vi "Read Asynchronous Measurement (Current and Voltage).vi"(6 "Wait Time (10 S)":u32=10, 7 "Voltage Buffer (smua.nvbuffer2)":string="smua.nvbuffer2", 8 "error in (no error)":errorcluster, 9 "Current Buffer (smua.nvbuffer1)":string="smua.nvbuffer1", 10 "Source Measure Unit Channel (0: Channel A)":i32(ring) items=["Channel A", "Channel B"], 11 "VISA resource name":refnum<visa-resource-name>) -> (0 "error out":errorcluster, 1 "Voltage Buffer Data (V)":dbl[](array[numeric]), 2 "Current Buffer Data (A)":dbl[](array[numeric]), 3 "VISA resource name out":refnum<visa-resource-name>)   [LabVIEW 2020, in "Keithley 2600 Series.lvlib"]
doc: "Returns the asynchronous current and voltage measurements."
uses:
  <instrlib>/Keithley 2600 Series/Keithley 2600 Series.lvlib
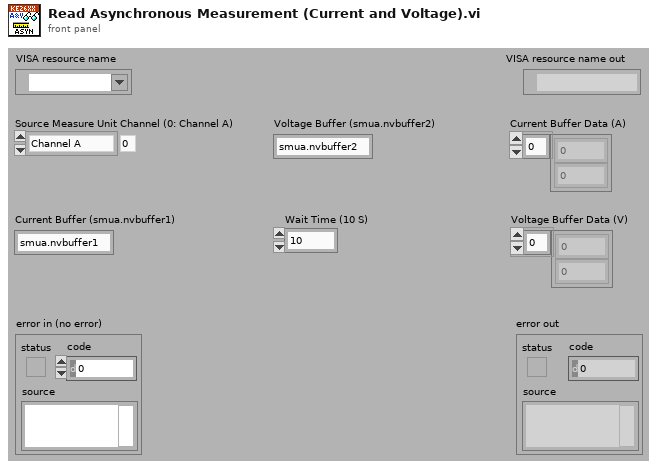
[diagram p1: front panel]
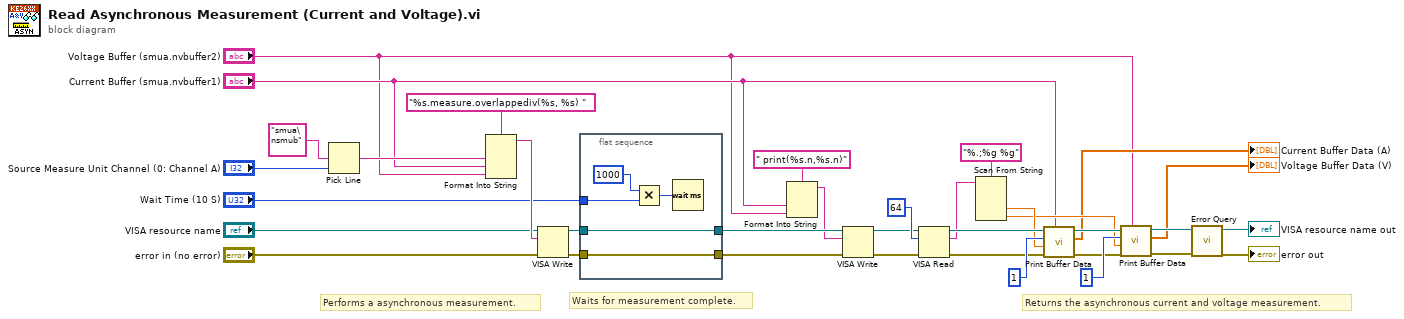
[diagram p0: block diagram]
diagram:
  # "Performs a asynchronous measurement."
  # "Waits for measurement complete."
  # "Returns the asynchronous current and voltage measurement."
  n1 = Pick Line(multi-line string="smua\nsmub", line index="Source Measure Unit Channel (0: Channel A)") -> (output string=w27:string)  [unwired: 1 in]
  n2 = Format Into String(format string="%s.measure.overlappediv(%s, %s) ", w27, "Current Buffer (smua.nvbuffer1)", "Voltage Buffer (smua.nvbuffer2)") -> (resulting string=w34:string)  [unwired: 2 in, 1 out]
  n3 = VISA Write(VISA resource name="VISA resource name", write buffer=w34, error in (no error)="error in (no error)") -> (VISA resource name out=w11:refnum<visa-resource-name>, error out=w10:errorcluster)  [unwired: 1 out]
  n4 = flat-sequence {
    tunnel: w11 -> [w40]
    tunnel: [w40] -> w8
    tunnel: [w39] -> w7
    tunnel: w10 -> [w39]
    tunnel: "Wait Time (10 S)" -> [w38]
    frame #0 {
      n5 = Multiply(x=u32 1000, y=w38) -> (x*y=w36:u32)
      n6 = Wait (ms)(milliseconds to wait=w36) -> ()  [unwired: 1 out]
    }
  }
  n7 = Format Into String(format string=" print(%s.n,%s.n)", "Current Buffer (smua.nvbuffer1)", "Voltage Buffer (smua.nvbuffer2)") -> (resulting string=w1:string)  [unwired: 2 in, 1 out]
  n8 = VISA Write(VISA resource name=w8, write buffer=w1, error in (no error)=w7) -> (VISA resource name out=w6:refnum<visa-resource-name>, error out=w5:errorcluster)  [unwired: 1 out]
  n9 = VISA Read(VISA resource name=w6, byte count=u32 64, error in (no error)=w5) -> (VISA resource name out=w24:refnum<visa-resource-name>, read buffer=w22:string, error out=w23:errorcluster)  [unwired: 1 out]
  n10 = Scan From String(format string="%.;%g %g", input string=w22) -> (output 1=w21:dbl, output 2=w14:dbl)  [unwired: 4 in, 3 out]
  n11 = call <instrlib>:"Print Buffer Data.vi"("Reading Buffer (smua.nvbuffer1)"="Current Buffer (smua.nvbuffer1)", "error in (no error)"=w23, "End Index (1)"=w21, "Start Index (1)"=1 ("Start Index (0)"), "VISA resource name"=w24) -> ("error out"=w17:errorcluster, "Buffer Data"=→"Current Buffer Data (A)":dbl[], "VISA resource name out"=w18:refnum<visa-resource-name>)  [unwired: 4 in]
  n12 = call <instrlib>:"Print Buffer Data.vi"("Reading Buffer (smua.nvbuffer1)"="Voltage Buffer (smua.nvbuffer2)", "error in (no error)"=w17, "End Index (1)"=w14, "Start Index (1)"=1 ("Start Index (0)"), "VISA resource name"=w18) -> ("error out"=w15:errorcluster, "Buffer Data"=→"Voltage Buffer Data (V)":dbl[], "VISA resource name out"=w16:refnum<visa-resource-name>)  [unwired: 4 in]
  n13 = call <instrlib>:"Error Query.vi"("error in (no error)"=w15, "VISA resource name"=w16) -> ("error out"=→"error out":errorcluster, "VISA resource name out"=→"VISA resource name out":refnum<visa-resource-name>)  [unwired: 6 in, 2 out]
